vi "VGD ECL AHMI PF SubVI02.vi"(0 "pixmap F":u32[][](array[numeric]), 5 "pixmap S":u32[][](array[numeric]), 7 "S":dbl=30.0 format="%#_13g", 9 "V":dbl=20.0 format="%#_13g", 11 "alfa":dbl[](array[slide]) scale=0.0..10.0) -> (4 "filas-1":i32, 6 "columnas-1":i32, 8 "pixmap COLOR":u32[][](array[numeric]), 10 "pixmap GF":u32[][](array[numeric]), 12 "Color":u32(colorbox), 15 "pixmap GS":u32[][](array[numeric]))   [LabVIEW 2020]
uses:
  <vilib>/picture/picture.llb/Draw True-Color Pixmap.vi
  <vilib>/Analysis/NI_AALBase.lvlib
panel:
  out "new picture":picture
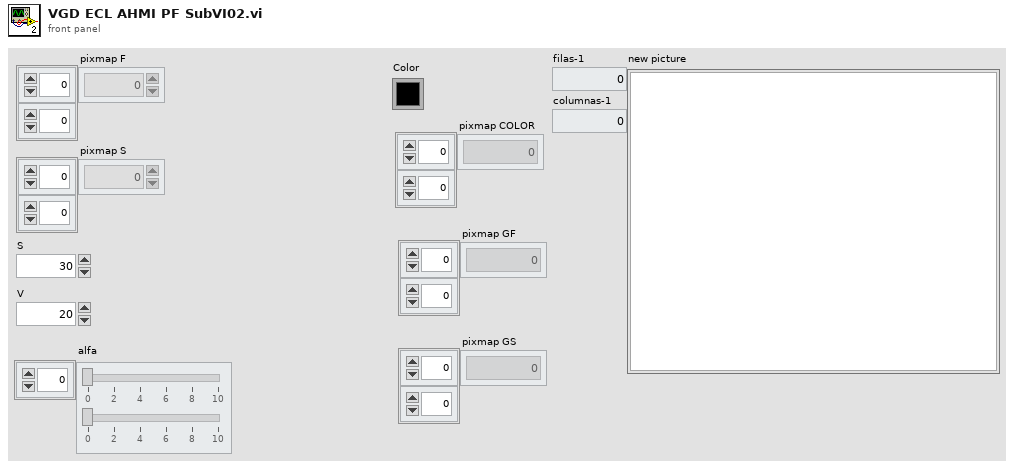
[diagram p1: front panel]
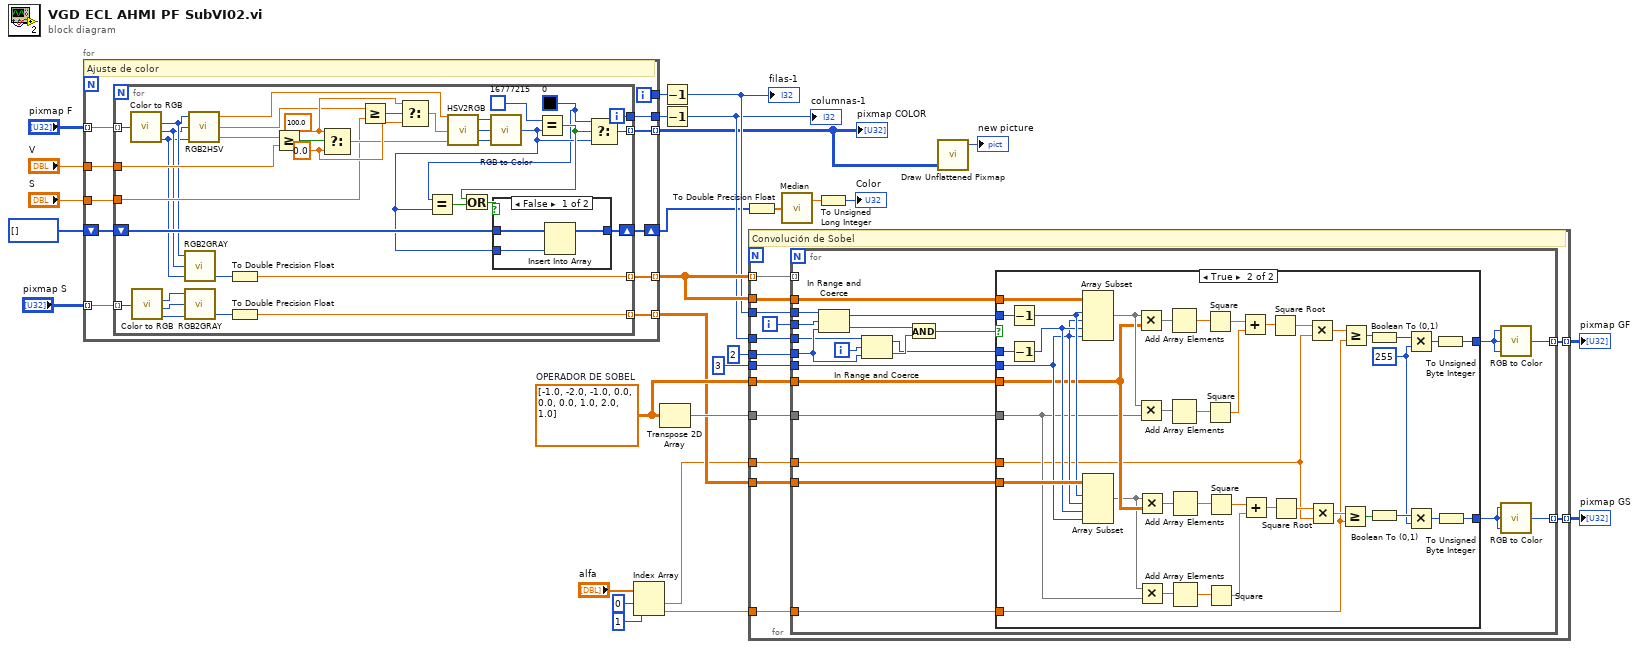
[diagram p0: block diagram]
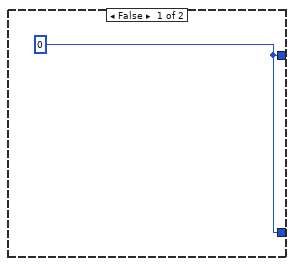
[diagram p2: hidden frame]
diagram:
  w20 = dbl[][] [[-1.0, -2.0, -1.0], [0.0, 0.0, 0.0], [1.0, 2.0, 1.0]]  # OPERADOR DE SOBEL
  n1 = for {
    tunnel: "pixmap F" -> [w39] mode=indexing
    tunnel: [w38] -> w2 mode=indexing
    tunnel: [w37] -> w17
    tunnel: [w36] -> w18
    tunnel: "V" -> [w35]
    tunnel: "S" -> [w34]
    shift-right: [w32] -> w10
    shift-left: u32[] [] -> [w33]
    tunnel: [w31] -> w19 mode=indexing
    tunnel: "pixmap S" -> [w30] mode=indexing
    tunnel: [w29] -> w14 mode=indexing
    i -> [w36]
    # "Ajuste de color"
    n2 = for {
      tunnel: w39 -> [w56] mode=indexing
      tunnel: [w64] -> w38 mode=indexing
      tunnel: [w63] -> w37
      tunnel: w35 -> [w62]
      tunnel: w34 -> [w61]
      shift-right: [w59] -> w32
      shift-left: w33 -> [w60]
      tunnel: [w51] -> w31 mode=indexing
      tunnel: w30 -> [w50] mode=indexing
      tunnel: [w45] -> w29 mode=indexing
      i -> [w63]
      w40 = u32 0
      w72 = 0.0 ("f")
      w73 = 100.0 ("t")
      n3 = call <vilib>:"Color to RGB.vi"("Color"=w56) -> ("R"=w55:u8, "G"=w54:u8, "B"=w53:u8)  [unwired: 1 out]
      n4 = call <vilib>:"Color to RGB.vi"("Color"=w50) -> ("R"=w47:u8, "G"=w48:u8, "B"=w49:u8)  [unwired: 1 out]
      n5 = call "RGB2GRAY.vi"("B"=w53, "G"=w54, "R"=w55) -> ("gray B"=w52:u8)  [unwired: 2 out]
      n6 = call "RGB2GRAY.vi"("B"=w49, "G"=w48, "R"=w47) -> ("gray B"=w46:u8)  [unwired: 2 out]
      n7 = call "RGB2HSV.vi"("B"=w53, "G"=w54, "R"=w55) -> ("V"=w57:dbl, "S"=w58:dbl, "H"=w69:dbl)
      n8 = To Double Precision Float(number=w52) -> (double precision float=w51:dbl)
      n9 = To Double Precision Float(number=w46) -> (double precision float=w45:dbl)
      n10 = Greater Or Equal?(x=w57, y=w62) -> (x >= y?=w75:bool)
      n11 = Select(t=w73, s=w75, f=w72) -> (s? t:f=w71:dbl)
      n12 = Greater Or Equal?(x=w58, y=w61) -> (x >= y?=w74:bool)
      n13 = Select(t=w73, s=w74, f=w72) -> (s? t:f=w70:dbl)
      n14 = call "HSV2RGB.vi"("V"=w71, "S"=w70, "H"=w69) -> ("B"=w66:u8, "G"=w67:u8, "R"=w68:u8)
      n15 = call <vilib>:"RGB to Color.vi"("B"=w66, "G"=w67, "R"=w68) -> ("Color"=w41:u32)
      n16 = Equal?(x=w40, y=w41) -> (x = y?=w44:bool)
      n17 = Equal?(x=u32 16777215, y=w41) -> (x = y?=w42:bool)
      n18 = Or(x=w42, y=w44) -> (x .or. y?=w43:bool)
      n19 = case shown="False" w43 {
        tunnel: w60 -> [w78 w79]
        tunnel: [w77 w79] -> w59
        tunnel: w41 -> [w76 _]
        frame False {
          n20 = Insert Into Array(array=w78, new element=w76) -> (w77:u32[])  [unwired: 1 in]
        }
        frame True {
        }
      }
      n21 = Select(t=w40, s=w42, f=w41) -> (s? t:f=w64:u32)
    }
  }
  "pixmap COLOR" <- w2
  n22 = Index Array(array="alfa", index #1=0 ("index"), index #2=1 ("index")) -> (element #1=w4:dbl, element #2=w3:dbl)
  n23 = Transpose 2D Array(2D array=w20) -> (transposed array=w21:dbl[][])
  n24 = Decrement(x=w18) -> (x-1=w16:i32)
  "filas-1" <- w16
  n25 = Decrement(x=w17) -> (x-1=w15:i32)
  "columnas-1" <- w15
  n26 = To Double Precision Float(number=w10) -> (double precision float=w11:dbl[])
  n27 = for {
    tunnel: w19 -> [w92] mode=indexing
    tunnel: w19 -> [w93]
    tunnel: w16 -> [w91]
    tunnel: w15 -> [w89]
    tunnel: [w88] -> w9 mode=indexing
    tunnel: 2 -> [w87]
    tunnel: 3 -> [w86]
    tunnel: w20 -> [w85]
    tunnel: w21 -> [w84]
    tunnel: w4 -> [w83]
    tunnel: w14 -> [w82]
    tunnel: [w81] -> w8 mode=indexing
    tunnel: w3 -> [w80]
    i -> [w90]
    # "Convolución de Sobel"
    n28 = for {
      tunnel: w93 -> [w106]
      tunnel: w91 -> [w114]
      tunnel: w89 -> [w112]
      tunnel: w87 -> [w113]
      tunnel: w86 -> [w103]
      tunnel: w90 -> [w111]
      tunnel: w85 -> [w102]
      tunnel: [w99] -> w88 mode=indexing
      tunnel: w92 -> [_] mode=indexing
      tunnel: w84 -> [w101]
      tunnel: w83 -> [w100]
      tunnel: w82 -> [w97]
      tunnel: [w96] -> w81 mode=indexing
      tunnel: w80 -> [w94]
      i -> [w110]
      n29 = In Range and Coerce(upper limit=w114, x=w111, lower limit=w113) -> (coerced(x)=w105:i32, In Range?=w109:bool)
      n30 = In Range and Coerce(upper limit=w112, x=w110, lower limit=w113) -> (coerced(x)=w104:i32, In Range?=w108:bool)
      n31 = And(x=w109, y=w108) -> (x .and. y?=w107:bool)
      n32 = case shown="True" w107 {
        tunnel: w106 -> [_ w153]
        tunnel: w105 -> [_ w155]
        tunnel: w104 -> [_ w154]
        tunnel: w103 -> [_ w139]
        tunnel: w102 -> [_ w130]
        tunnel: [w115 w143] -> w98
        tunnel: w101 -> [_ w128]
        tunnel: w100 -> [_ w127]
        tunnel: w97 -> [_ w142]
        tunnel: [w115 w126] -> w95
        tunnel: w94 -> [_ w123]
        frame False {
          w115 = u8 0
        }
        frame True {
          w118 = i16 255 ("y")
          n33 = Decrement(x=w155) -> (x-1=w141:i32)
          n34 = Decrement(x=w154) -> (x-1=w140:i32)
          n35 = Array Subset(array=w153, index (row)=w141, length (row)=w139, index (col)=w140, length (col)=w139) -> (w151:dbl[][])
          n36 = Array Subset(array=w142, index (row)=w141, length (row)=w139, index (col)=w140, length (col)=w139) -> (w129:dbl[][])
          n37 = Multiply(x=w151, y=w130) -> (x*y=w152:dbl[][])
          n38 = Multiply(x=w151, y=w128) -> (x*y=w150:dbl[][])
          n39 = Multiply(x=w129, y=w130) -> (x*y=w131:dbl[][])
          n40 = Multiply(x=w129, y=w128) -> (x*y=w132:dbl[][])
          n41 = Add Array Elements(numeric array=w152) -> (sum=w149:dbl)
          n42 = Add Array Elements(numeric array=w150) -> (sum=w148:dbl)
          n43 = Add Array Elements(numeric array=w131) -> (sum=w133:dbl)
          n44 = Add Array Elements(numeric array=w132) -> (sum=w134:dbl)
          n45 = Square(x=w149) -> (x^2=w147:dbl)
          n46 = Square(x=w148) -> (x^2=w146:dbl)
          n47 = Square(x=w133) -> (x^2=w135:dbl)
          n48 = Square(x=w134) -> (x^2=w136:dbl)
          n49 = Add(x=w147, y=w146) -> (x+y=w145:dbl)
          n50 = Add(x=w135, y=w136) -> (x+y=w137:dbl)
          n51 = Square Root(x=w145) -> (sqrt(x)=w144:dbl)
          n52 = Square Root(x=w137) -> (sqrt(x)=w138:dbl)
          n53 = Multiply(x=w144, y=w127) -> (x*y=w125:dbl)
          n54 = Multiply(x=w138, y=w127) -> (x*y=w124:dbl)
          n55 = Greater Or Equal?(x=w124, y=w123) -> (x >= y?=w121:bool)
          n56 = Greater Or Equal?(x=w125, y=w123) -> (x >= y?=w122:bool)
          n57 = Boolean To (0,1)(Boolean=w122) -> (0, 1=w120:i16)
          n58 = Boolean To (0,1)(Boolean=w121) -> (0, 1=w119:i16)
          n59 = Multiply(x=w120, y=w118) -> (x*y=w117:i16)
          n60 = Multiply(x=w119, y=w118) -> (x*y=w116:i16)
          n61 = To Unsigned Byte Integer(number=w117) -> (unsigned 8bit integer=w143:u8)
          n62 = To Unsigned Byte Integer(number=w116) -> (unsigned 8bit integer=w126:u8)
        }
      }
      n63 = call <vilib>:"RGB to Color.vi"("B"=w98, "G"=w98, "R"=w98) -> ("Color"=w99:u32)
      n64 = call <vilib>:"RGB to Color.vi"("B"=w95, "G"=w95, "R"=w95) -> ("Color"=w96:u32)
    }
  }
  "pixmap GF" <- w9
  "pixmap GS" <- w8
  n65 = call <vilib>:"Median.vi"("X"=w11) -> ("median"=w13:dbl)  [unwired: 1 out]
  n66 = To Unsigned Long Integer(number=w13) -> (unsigned 32bit integer=→"Color":u32)
  n67 = call-poly <vilib>:"Draw Unflattened Pixmap.vi"("data (RGB format)"=w2) -> ("new picture"=→"new picture":picture)  [unwired: 8 in]
